vi "DAQmx for current integrator.vi"() -> ()   [LabVIEW 2011]
uses:
  <vilib>/DAQmx/write.llb/DAQmx Write (Digital Bool 1Line 1Point).vi
  <vilib>/DAQmx/read.llb/DAQmx Read (Analog 1D DBL 1Chan NSamp).vi
  <vilib>/DAQmx/create/channels.llb/DAQmx Create Channel (AI-Voltage-Basic).vi
  <vilib>/DAQmx/configure/timing.llb/DAQmx Timing (Sample Clock).vi
  <vilib>/DAQmx/configure/trigger.llb/DAQmx Start Trigger (Digital Edge).vi
  <vilib>/DAQmx/create/channels.llb/DAQmx Create Channel (DO-Digital Output).vi
  <vilib>/DAQmx/create/channels.llb/DAQmx Create Channel (CO-Pulse Generation-Time).vi
  <vilib>/DAQmx/configure/timing.llb/DAQmx Timing (Implicit).vi
  <vilib>/DAQmx/miscellaneous.llb/DAQmx Fill In Error Info.vi
panel:
  out "data":dbl[](array[numeric])=[1.151598858, 1.3161641700000002, 1.3624481640000001, 1.3778761620000002, 1.413874824, 1.4447308200000002, 1.47044415, 1.4910148140000001, 1.5218708100000002, 1.542441474, 1.5681548040000002, 1.3007361720000001, 1.275022842, 1.2647375100000002, 1.228738848, 1.218453516, 1.2030255180000002, 1.1875975200000002, 1.1721695220000001, 1.16188419, 1.156741524, 1.3264495020000002, 1.347020166, 1.3984468260000003, 1.413874824, 1.4498734860000002, 1.47044415, 1.4961574800000002, 1.5167281440000002, 1.537298808, 1.5681548040000002, 1.3110215040000002, 1.280165508, 1.2493095120000002, 1.2338815140000001, 1.21331085, 1.1978828520000002, 1.1875975200000002, 1.156741524, 1.156741524, 1.141313526, 1.3315921680000002, 1.357305498, 1.3778761620000002, 1.413874824, 1.4498734860000002, 1.47044415, 1.4961574800000002, 1.5270134760000003, 1.54758414, 1.5630121380000002, 1.3110215040000002, 1.285308174, 1.2493095120000002, 1.2390241800000001, 1.208168184, 1.2030255180000002, 1.1670268560000001, 1.1773121880000001, 1.1721695220000001, 1.151598858, 1.3264495020000002, 1.357305498, 1.3830188280000002, 1.413874824, 1.4447308200000002, 1.47044415, 1.4910148140000001, 1.5218708100000002, 1.542441474, 1.5630121380000002, 1.3110215040000002, 1.2698801760000002, 1.2441668460000002, 1.2390241800000001, 1.21331085, 1.1978828520000002, 1.1824548540000002, 1.1670268560000001, 1.156741524, 1.151598858, 1.3213068360000002, 1.357305498, 1.3778761620000002, 1.41901749, 1.4498734860000002, 1.47044415, 1.4961574800000002, 1.5218708100000002, 1.542441474, 1.5578694720000001, 1.3058788380000002, 1.2698801760000002, 1.2493095120000002, 1.2338815140000001, 1.2030255180000002, 1.1875975200000002, 1.1875975200000002, 1.1721695220000001, 1.16188419] format="%0.2f"
  in  "V0 units":i32(ring)=10348 items=["Volts"=10348, "From Custom Scale"=10065]
  in  "minimum value":dbl=-5.0 format="%0.2f"
  in  "maximum value":dbl=5.0 format="%0.2f"
  in  "input terminal configuration":i32(ring)=-1 items=["default"=-1, "RSE"=10083, "NRSE"=10078, "Differential"=10106, "Pseudodifferential"=12529]
  in  "V0":tag="cDAQ1Mod1/ai0"
  in  "S1":tag="cDAQ1Mod5/port0/line4"
  in  "sample mode":i32(ring)=10123 items=["Finite Samples"=10178, "Continuous Samples"=10123, "Hardware Timed Single Point"=12522]
  out "error out":errorcluster
  in  "initial delay":dbl format="%.6f"
  in  "S2 units":i32(ring)=10364 items=["Seconds"=10364]
  in  "low time":dbl=1e-05 format="%.6f"
  in  "high time":dbl=0.00999 format="%.6f"
  in  "S2":tag="cDAQ1Mod5/ctr0"
  in  "stop":bool
  in  "error in":errorcluster
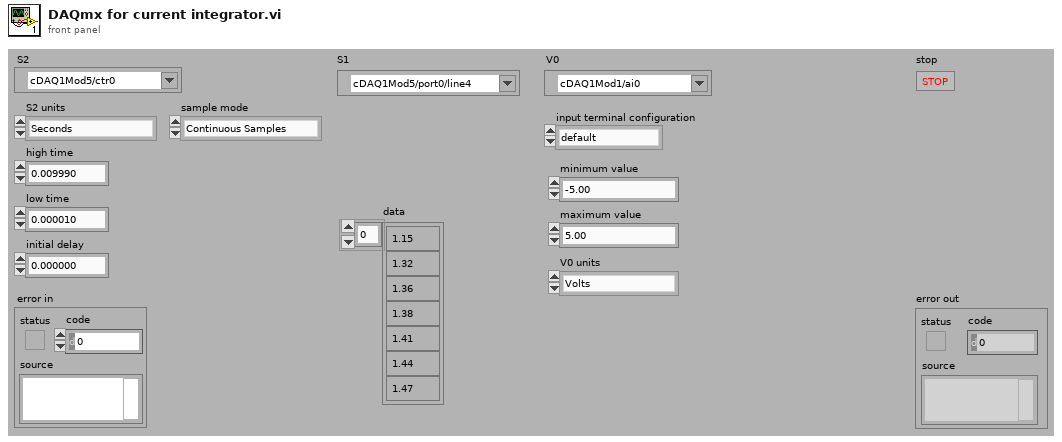
[diagram p1: front panel]
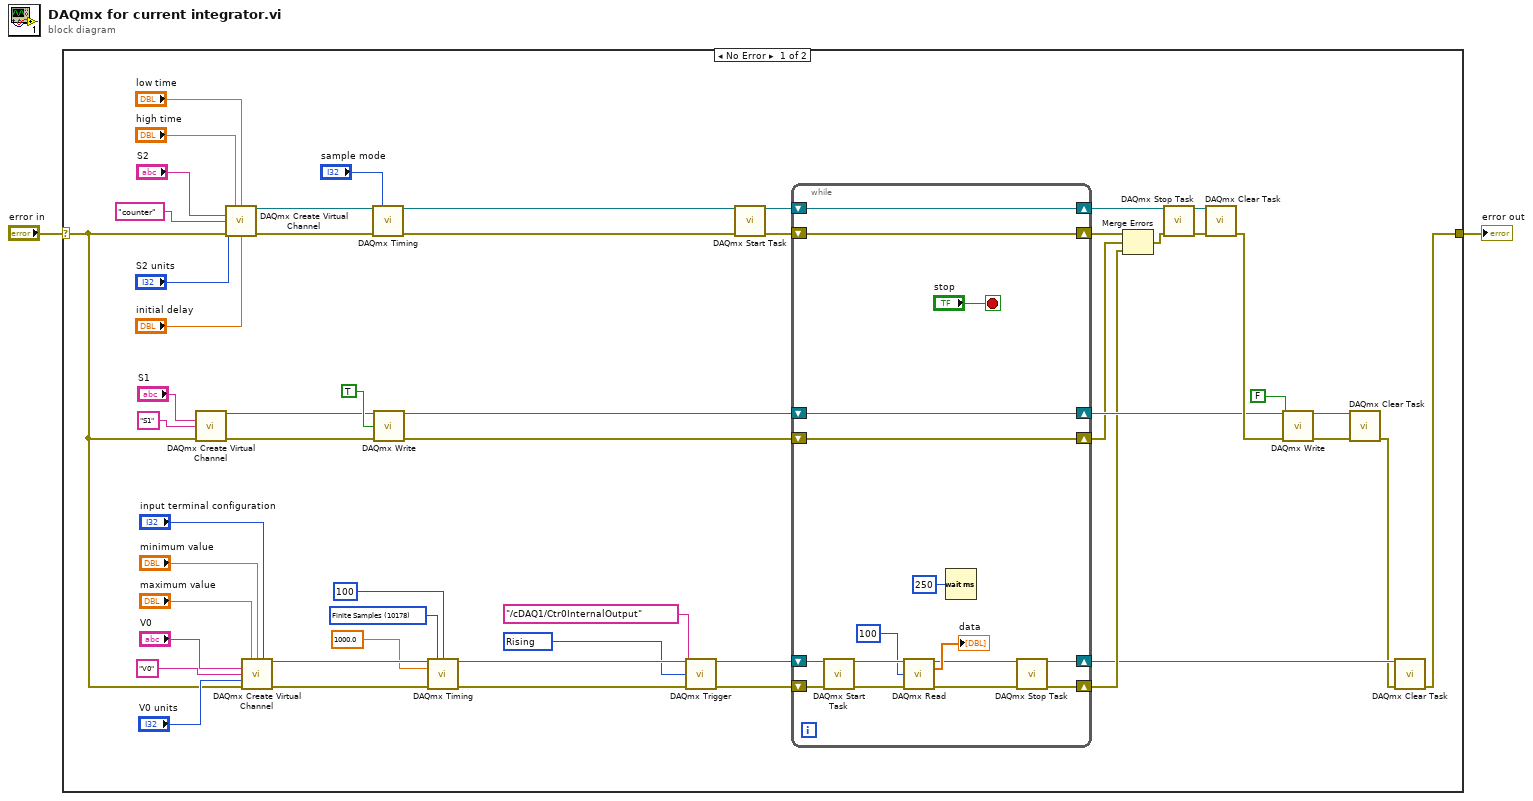
[diagram p0: block diagram]
diagram:
  n1 = case shown="No Error" "error in" {
    selector: "error in" -> [w30 w72]
    tunnel: [w39 w72] -> w2
    frame No Error {
      w17 = 10280 items=["Rising"=10280, "Falling"=10171] ("edge")
      w32 = 10178 items=["Finite Samples"=10178, "Continuous Samples"=10123, "Hardware Timed Single Point"=12522] ("sample mode")
      n2 = call-poly <vilib>:"DAQmx Create Virtual Channel.vi"("lines"="S1", "name to assign"="S1", "error in"=w30) -> ("task out"=w27:refnum<k21>, "error out"=w28:errorcluster)  [unwired: 11 in]
      n3 = call-poly <vilib>:"DAQmx Create Virtual Channel.vi"("high time"="high time", "low time"="low time", "counter"="S2", "name to assign"="counter", "units"="S2 units", "error in"=w30, "initial delay"="initial delay") -> ("task out"=w53:refnum<k21>, "error out"=w52:errorcluster)  [unwired: 7 in]
      n4 = call-poly <vilib>:"DAQmx Create Virtual Channel.vi"("maximum value"="maximum value", "minimum value"="minimum value", "input terminal configuration"="input terminal configuration", "physical channels"="V0", "name to assign"="V0", "units"="V0 units", "error in"=w30) -> ("task out"=w37:refnum<k21>, "error out"=w38:errorcluster)  [unwired: 7 in]
      n5 = call-poly <vilib>:"DAQmx Timing.vi"("task/channels in"=w53, "sample mode"="sample mode", "error in"=w52) -> ("task out"=w23:refnum<k21>, "error out"=w21:errorcluster)  [unwired: 11 in]
      n6 = call-poly <vilib>:"DAQmx Write.vi"("task/channels in"=w27, "data"=TRUE, "error in"=w28) -> ("task out"=w9:refnum<k21>, "error out"=w7:errorcluster)  [unwired: 10 in, 1 out]
      n7 = call-poly <vilib>:"DAQmx Timing.vi"("task/channels in"=w37, "sample mode"=w32, "samples per channel"=100, "rate"=1000.0, "error in"=w38) -> ("task out"=w19:refnum<k21>, "error out"=w18:errorcluster)  [unwired: 9 in]
      n8 = call-poly <vilib>:"DAQmx Trigger.vi"("task/channels in"=w19, "source"=tag "/cDAQ1/Ctr0InternalOutput", "edge"=w17, "error in"=w18) -> ("task out"=w15:refnum<k21>, "error out"=w14:errorcluster)  [unwired: 10 in]
      n9 = call <vilib>:"DAQmx Start Task.vi"("task/channels in"=w23, "error in"=w21) -> ("task out"=w13:refnum<k21>, "error out"=w12:errorcluster)  [unwired: 12 in]
      n10 = while {
        shift-right: [w64] -> w11
        shift-left: w13 -> [w64]
        shift-right: [w65] -> w10
        shift-left: w12 -> [w65]
        shift-right: [w63] -> w8
        shift-left: w9 -> [w63]
        shift-right: [w62] -> w6
        shift-left: w7 -> [w62]
        shift-right: [w57] -> w4
        shift-left: w15 -> [w70]
        shift-right: [w56] -> w5
        shift-left: w14 -> [w69]
        stop <- "stop" stop-if-true
        n11 = call <vilib>:"DAQmx Start Task.vi"("task/channels in"=w70, "error in"=w69) -> ("task out"=w71:refnum<k21>, "error out"=w61:errorcluster)  [unwired: 12 in]
        n12 = call-poly <vilib>:"DAQmx Read.vi"("task/channels in"=w71, "number of samples per channel"=100, "error in"=w61) -> ("task out"=w59:refnum<k21>, "data"=→"data":dbl[], "error out"=w58:errorcluster)  [unwired: 10 in]
        n13 = Wait (ms)(milliseconds to wait=u32 250) -> ()  [unwired: 1 out]
        n14 = call <vilib>:"DAQmx Stop Task.vi"("task/channels in"=w59, "error in"=w58) -> ("task out"=w57:refnum<k21>, "error out"=w56:errorcluster)  [unwired: 12 in]
      }
      n15 = Merge Errors(w10, w6, w5) -> (w22:errorcluster)
      n16 = call <vilib>:"DAQmx Stop Task.vi"("task/channels in"=w11, "error in"=w22) -> ("task out"=w55:refnum<k21>, "error out"=w54:errorcluster)  [unwired: 12 in]
      n17 = call <vilib>:"DAQmx Clear Task.vi"("task in"=w55, "error in"=w54) -> ("error out"=w33:errorcluster)  [unwired: 13 in]
      n18 = call-poly <vilib>:"DAQmx Write.vi"("task/channels in"=w8, "data"=FALSE, "error in"=w33) -> ("task out"=w34:refnum<k21>, "error out"=w35:errorcluster)  [unwired: 10 in, 1 out]
      n19 = call <vilib>:"DAQmx Clear Task.vi"("task in"=w34, "error in"=w35) -> ("error out"=w3:errorcluster)  [unwired: 13 in]
      n20 = call <vilib>:"DAQmx Clear Task.vi"("task in"=w4, "error in"=w3) -> ("error out"=w39:errorcluster)  [unwired: 13 in]
    }
    frame Error {
    }
  }
  "error out" <- w2
